vi "Cull and Group.vi"(9 "Score Cutoff":dbl=70.0, 10 "Sorted Data":dbl[][](array[numeric])) -> (0 "Rect":T1, 1 "Line":T1, 2 "Score":dbl, 3 "Center":cluster{"X":dbl, "Y":dbl})   [LabVIEW 2016]
doc: "Examine the particle measurements to find the most likely pair that make up the target. This mostly compares the edges of the bounding boxes. It then returns information about the overall target, notably the rectangle sourrounding the particles, the vertical line that bisects the target, and the center of the top particle."
panel:
  out "Grouping Scores":T2(array[cluster])
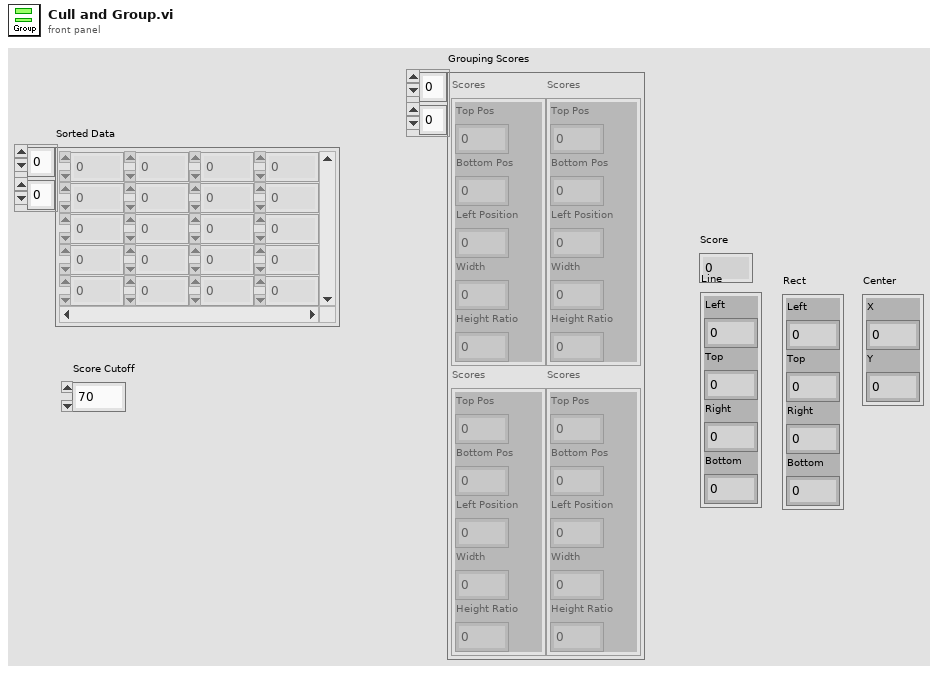
[diagram p1: front panel]
types:
  T1 = cluster{"Left":dbl, "Top":dbl, "Right":dbl, "Bottom":dbl}
  T2 = cluster{"Top Pos":dbl, "Bottom Pos":dbl, "Left Position":dbl, "Width":dbl, "Height Ratio":dbl}[][]
  T3 = cluster{"Top Position":dbl, "Bottom Position":dbl, "Left Gap":dbl, "Width":dbl, "Height Ratio":dbl}
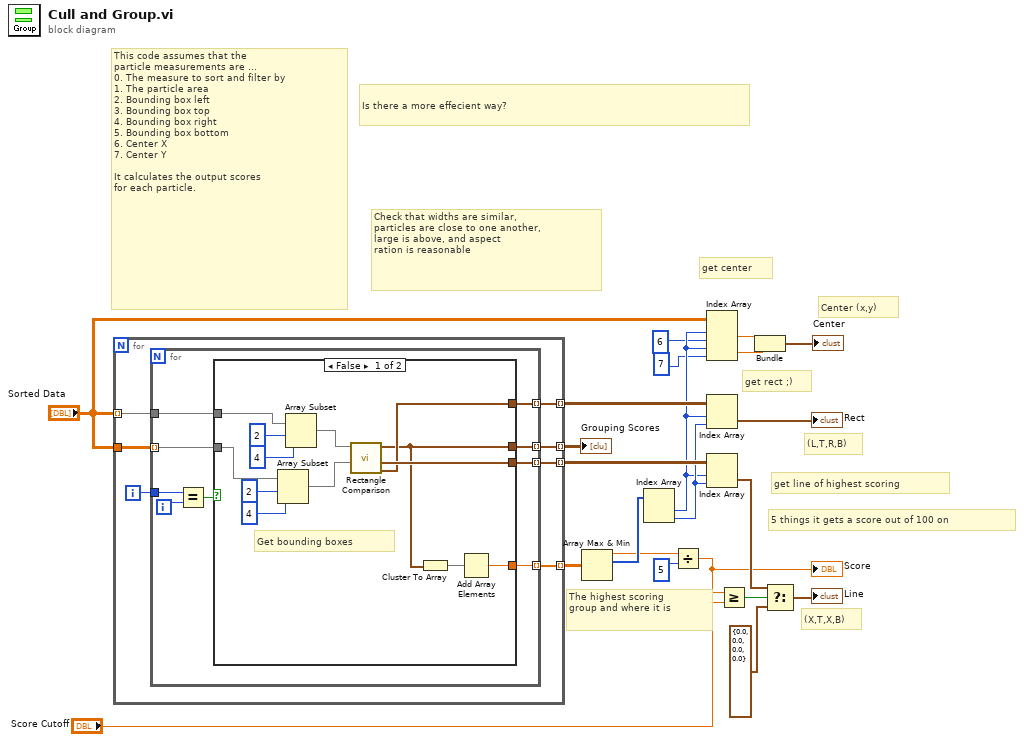
[diagram p0: block diagram]
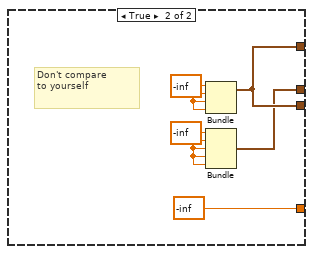
[diagram p2: hidden frame]
diagram:
  # "Is there a more effecient way?"
  # "5 things it gets a score out of 100 on"
  # "get center"
  # "get rect ;)"
  # "get line of highest scoring"
  # "The highest scoring\ngroup and where it is"
  # "(X,T,X,B)"
  # "(L,T,R,B)"
  # "Center (x,y)"
  # "Check that widths are similar,\nparticles are close to one another,\nlarge is above, and aspect\nration is reasonable"
  # "This code assumes that the\nparticle measurements are ...\n0. The measure to sort and filter by\n1. The particle area\n2. Bounding box left\n3. Bounding box top\n4. Bounding box right\n5. Bounding box bottom\n6. Center X\n7. Center Y\n\nIt calculates the output scores\nfor each particle."
  n1 = for {
    tunnel: "Sorted Data" -> [w29] mode=indexing
    tunnel: "Sorted Data" -> [w28]
    tunnel: [w27] -> w22 mode=indexing
    tunnel: [w25] -> w21 mode=indexing
    tunnel: [w24] -> w18 mode=indexing
    tunnel: [w23] -> w14 mode=indexing
    i -> [w26]
    n2 = for {
      tunnel: w29 -> [w38]
      tunnel: w28 -> [w36] mode=indexing
      tunnel: [w35] -> w27 mode=indexing
      tunnel: w26 -> [w34]
      tunnel: [w32] -> w25 mode=indexing
      tunnel: [w31] -> w24 mode=indexing
      tunnel: [w30] -> w23 mode=indexing
      i -> [w33]
      n3 = Equal?(x=w34, y=w33) -> (x = y?=w37:bool)
      n4 = case shown="False" w37 {
        tunnel: w38 -> [w49 _]
        tunnel: w36 -> [w46 _]
        tunnel: [w39 w52] -> w35
        tunnel: [w44 -inf] -> w32
        tunnel: [w41 w55] -> w31
        tunnel: [w40 w55] -> w30
        frame False {
          # "Get bounding boxes"
          n5 = Array Subset(array=w46, index=2, length=4) -> (w42:dbl[])
          n6 = Array Subset(array=w49, index=2, length=4) -> (w43:dbl[])
          n7 = call "Rectangle Comparison.vi"("Second"=w42, "First"=w43) -> ("Rect"=w40:T1, "Line"=w41:T1, "Scores"=w39:T3)  [unwired: 7 in]
          n8 = Cluster To Array(cluster=w39) -> (array=w45:dbl[])
          n9 = Add Array Elements(numeric array=w45) -> (sum=w44:dbl)
        }
        frame True {
          w53 = -inf
          w54 = -inf
          # "Don't compare\nto yourself"
          n10 = Bundle(w54, w54, w54, w54) -> (w55:cluster{dbl, dbl, dbl, dbl})  [unwired: 1 in]
          n11 = Bundle(w53, w53, w53, w53, w53) -> (w52:cluster{dbl, dbl, dbl, dbl, dbl})  [unwired: 1 in]
        }
      }
    }
  }
  "Grouping Scores" <- w22
  n12 = Array Max & Min(array=w21) -> (max value=w3:dbl, max index (indices)=w4:i32[])  [unwired: 2 out]
  n13 = Index Array(array=w4) -> (element #1=w10:i32, element #2=w13:i32)  [unwired: 2 in]
  n14 = Divide(x=w3, y=5 ("length")) -> (x/y=w2:dbl)
  "Score" <- w2
  n15 = Index Array(array="Sorted Data", index (row) #1=w10, index (col) #1=6 ("index"), index (row) #2=w10, index (col) #2=7 ("index")) -> (element #1=w8:dbl, element #2=w7:dbl)
  n16 = Index Array(array=w14, index (row)=w10, index (col)=w13) -> (element=→"Rect":T1)
  n17 = Index Array(array=w18, index (row)=w10, index (col)=w13) -> (element=w17:T1)
  n18 = Greater Or Equal?(x=w2, y="Score Cutoff") -> (x >= y?=w20:bool)
  n19 = Bundle("Numeric"=w8, "Numeric"=w7) -> (→"Center":cluster{"Numeric":dbl, "Numeric":dbl})  [unwired: 1 in]
  n20 = Select(t=w17, s=w20, f=cluster{dbl, "Top":dbl, dbl, "Bottom":dbl} {0.0, "Top"=0.0, 0.0, "Bottom"=0.0}) -> (s? t:f=→"Line":T1)
